vi "zad3.vi"() -> ()   [LabVIEW 2017]
panel:
  in  "stop":bool
  out "Numeric":dbl
  in  "K":i64
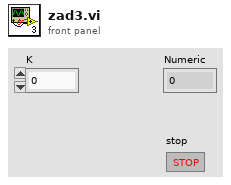
[diagram p1: front panel]
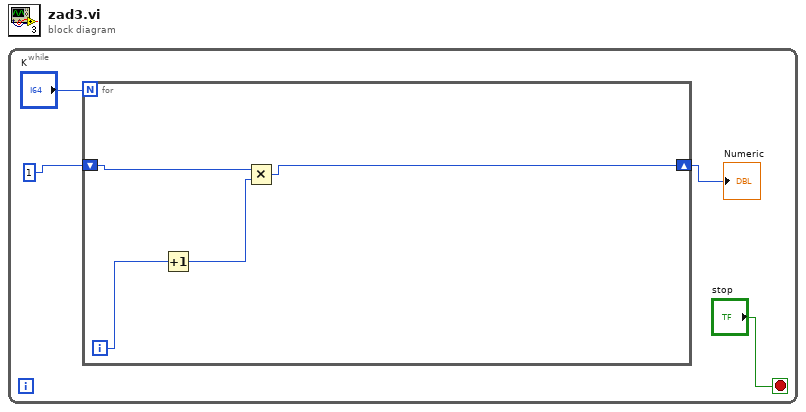
[diagram p0: block diagram]
diagram:
  n1 = while {
    stop <- "stop" stop-if-true
    n2 = for {
      N: "K" -> [_]
      shift-right: [w5] -> w1
      shift-left: i64 1 ("Numeric") -> [w6]
      i -> [w8]
      n3 = Increment(x=w8) -> (x+1=w7:i32)
      n4 = Multiply(x=w6, y=w7) -> (x*y=w5:i64)
    }
    "Numeric" <- w1
  }
